vi "boolean.vi"() -> ()   [LabVIEW 2020]
uses:
  <vilib>/Utility/miscctls.llb/LVPositionTypeDef.ctl
panel:
  out "Position":T1
  out "Boolean":bool
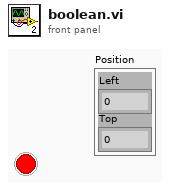
[diagram p1: front panel]
types:
  T1 = typedef "LVPositionTypeDef.ctl" = cluster{"Left":i32, "Top":i32}
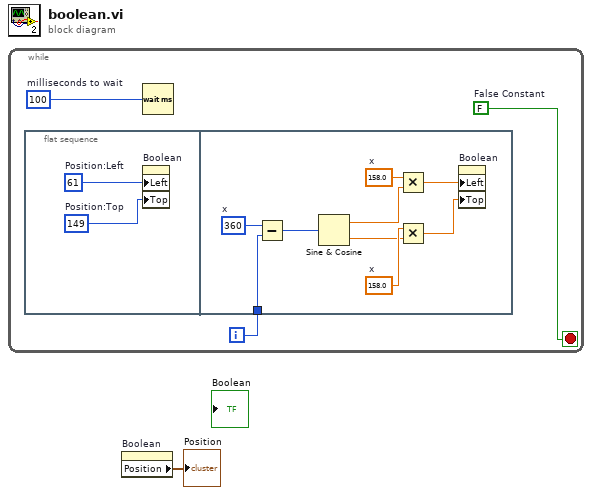
[diagram p0: block diagram]
diagram:
  n1 = while {
    i -> [w2]
    stop <- w3 stop-if-true
    w3 = FALSE  # False Constant
    w4 = u32 100  # milliseconds to wait
    n2 = flat-sequence {
      tunnel: w2 -> [w14]
      frame #0 {
        w5 = 149  # Position:Top
        w6 = 61  # Position:Left
        n3 = property on="Boolean" class="Bool (strict)"("Left"=w6, "Top"=w5) -> ()  [unwired: 2 in, 2 out]
      }
      frame #1 {
        w10 = 158.0  # x
        w11 = 158.0  # x
        w15 = 360  # x
        n4 = Subtract(x=w15, y=w14) -> (x-y=w13:i32)
        n5 = Sine & Cosine(0:w13) -> (1:w12:dbl, 2:w9:dbl)
        n6 = Multiply(x=w11, y=w12) -> (x*y=w8:dbl)
        n7 = Multiply(x=w10, y=w9) -> (x*y=w7:dbl)
        n8 = property on="Boolean" class="Bool (strict)"("Left"=w8, "Top"=w7) -> ()  [unwired: 2 in, 2 out]
      }
    }
    n9 = Wait (ms)(milliseconds to wait=w4) -> ()  [unwired: 1 out]
  }
  n10 = property on="Boolean" class="Bool (strict)"() -> ("Position"=→"Position":T1)  [unwired: 2 in, 2 out]
